vi "Read Row.vi"(8 "error in (no error)":errorcluster, 11 "UserAddedRow in":refnum<class "UserAddedRow.lvclass">) -> (0 "error out":errorcluster, 2 "Row":refnum<k24>, 3 "UserAddedRow out":refnum<class "UserAddedRow.lvclass">)   [LabVIEW 2014, in "DataGrid.lvlib" / "UserAddedRow.lvclass"]
uses:
  UserAddedRow.lvclass
  System.Windows.Forms
  UserAddedRow.lvclass/UserAddedRow.ctl
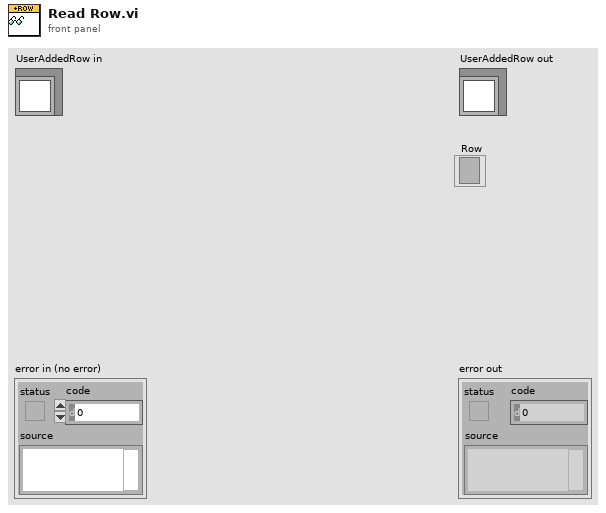
[diagram p1: front panel]
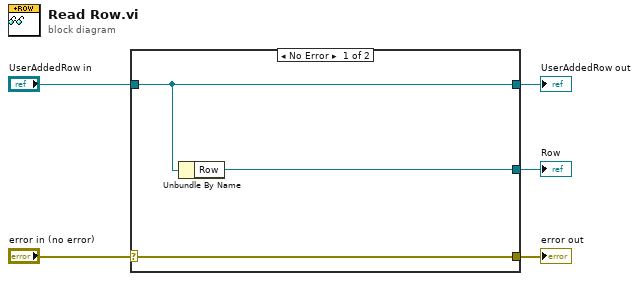
[diagram p0: block diagram]
diagram:
  n1 = case shown="No Error" "error in (no error)" {
    selector: "error in (no error)" -> [w8 w9]
    tunnel: [w8 w9] -> w4
    tunnel: [w7 w10] -> w2
    tunnel: "UserAddedRow in" -> [w7 w10]
    tunnel: [w6 _] -> w1
    frame No Error {
      n2 = Unbundle By Name(w7) -> ("Row"=w6:refnum<k24>)
    }
    frame Error {
    }
  }
  "error out" <- w4
  "UserAddedRow out" <- w2
  "Row" <- w1
